vi "add_time.vi"   [LabVIEW 2010]
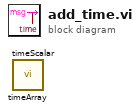
[diagram p0: block diagram]
diagram:
  n1 = call <userlib>:"timeArray.vi"() -> ()  [unwired: 5 in, 1 out]
  n2 = call <userlib>:"timeScalar.vi"() -> ()  [unwired: 5 in, 1 out]
